vi "APC_9049_HRL_preChamber.vi"(2 "InCylPressure":dbl[](array[numeric]), 3 "PrechamberPressure":dbl[](array[numeric])) -> (0 "peakPrechamberPdiff":dbl, 1 "PreIgnition":bool)   [LabVIEW 2020]
panel:
  in  "PeggingWindowsLength [samples]":i32=200
  in  "PeggingWindowStart [samples]":i32=2500
  out "Residuum":dbl[](graph)
  in  "threshold [bar]":dbl=5.0 format="%#_13g"
  in  "PeakCalculationWindowLength [samples]":i32=600
  in  "PeakCalculationWindowStart [samples]":i32=3000
  in  "Graph?":bool
  out "Pressure pegging":dbl[][](graph)
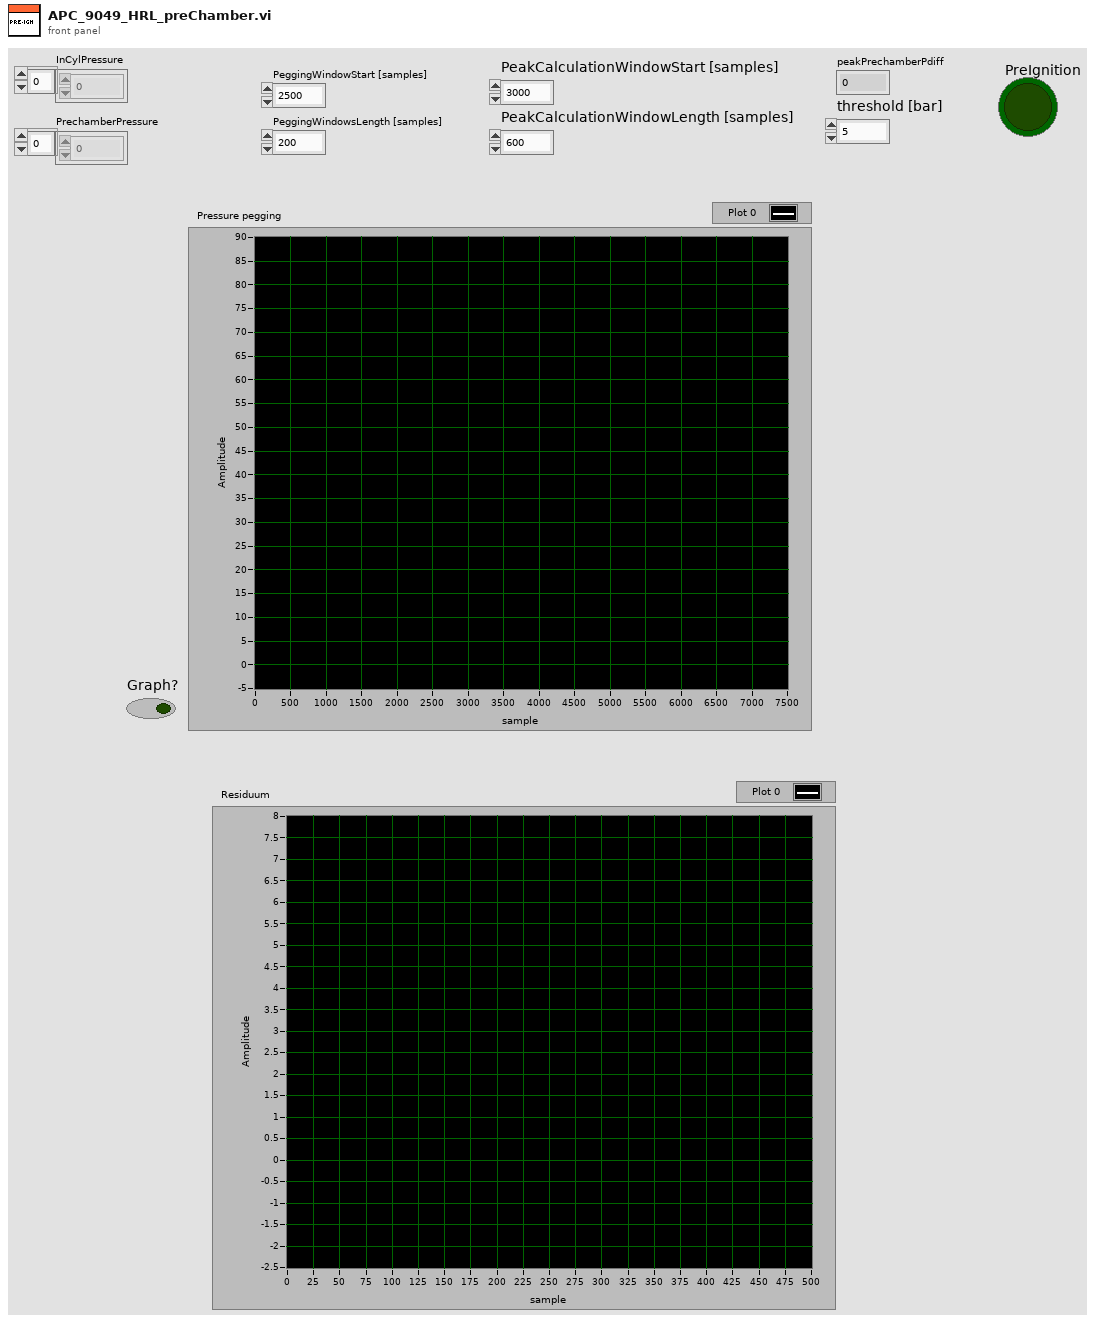
[diagram p1: front panel]
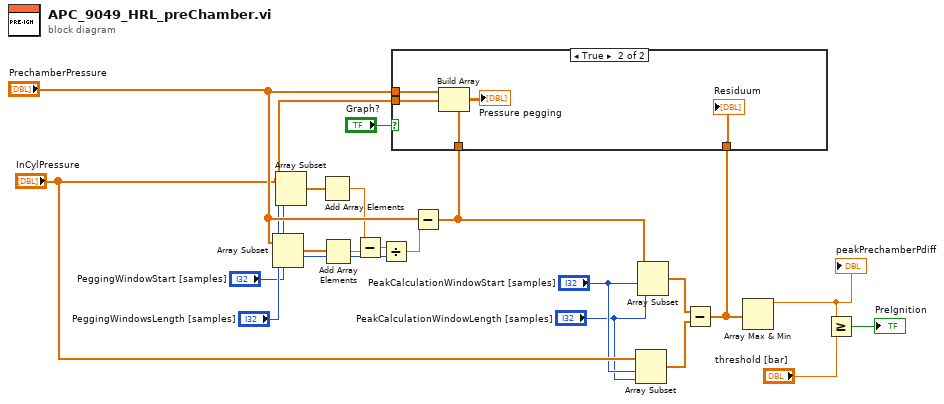
[diagram p0: block diagram]
diagram:
  n1 = Array Subset(array="PrechamberPressure", index="PeggingWindowStart [samples]", length="PeggingWindowsLength [samples]") -> (w12:dbl[])
  n2 = Array Subset(array="InCylPressure", index="PeggingWindowStart [samples]", length="PeggingWindowsLength [samples]") -> (w14:dbl[])
  n3 = Add Array Elements(numeric array=w14) -> (sum=w16:dbl)
  n4 = Add Array Elements(numeric array=w12) -> (sum=w15:dbl)
  n5 = Subtract(x=w15, y=w16) -> (x-y=w17:dbl)
  n6 = Divide(x=w17, y="PeggingWindowsLength [samples]") -> (x/y=w19:dbl)
  n7 = Subtract(x="PrechamberPressure", y=w19) -> (x-y=w10:dbl[])
  n8 = Array Subset(array="InCylPressure", index="PeakCalculationWindowStart [samples]", length="PeakCalculationWindowLength [samples]") -> (w5:dbl[])
  n9 = Array Subset(array=w10, index="PeakCalculationWindowStart [samples]", length="PeakCalculationWindowLength [samples]") -> (w6:dbl[])
  n10 = Subtract(x=w6, y=w5) -> (x-y=w2:dbl[])
  n11 = case shown="True" "Graph?" {
    tunnel: "InCylPressure" -> [_ w25]
    tunnel: w10 -> [_ w24]
    tunnel: "PrechamberPressure" -> [_ w23]
    tunnel: w2 -> [_ w21]
    frame False {
    }
    frame True {
      n12 = Build Array(w23, w25, w24) -> (→"Pressure pegging":dbl[][])
      "Residuum" <- w21
    }
  }
  n13 = Array Max & Min(array=w2) -> (max value=w1:dbl)  [unwired: 3 out]
  "peakPrechamberPdiff" <- w1
  n14 = Greater Or Equal?(x=w1, y="threshold [bar]") -> (x >= y?=→"PreIgnition":bool)
